vi "FunctDataMgr.Send Local SW Info.vi"(8 "error in (no error)":errorcluster, 11 "FunctDataMgr in":refnum<class "FunctDataMgr.lvclass">) -> (0 "error out":errorcluster, 3 "FunctDataMgr out":refnum<class "FunctDataMgr.lvclass">)   [LabVIEW 2018, in "FunctDataMgr.lvclass"]
uses:
  FunctDataMgr.lvclass
  FunctDataMgr.lvclass/FunctDataMgr.ctl
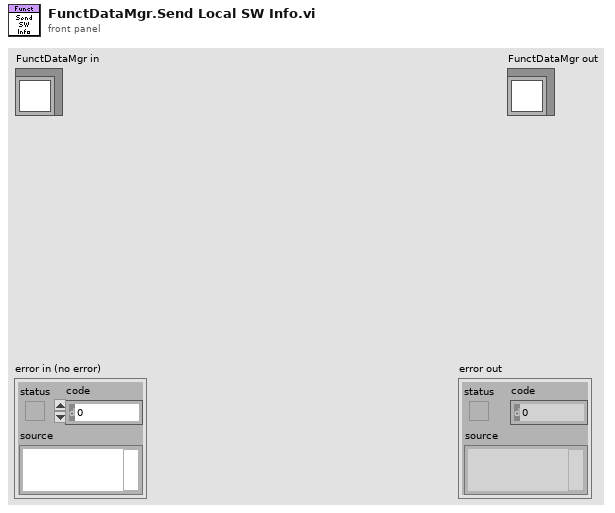
[diagram p1: front panel]
types:
  T1 = typedef "TestResult.SW Item.ctl" = cluster{"Name":string, "PN":string, "Version":string, "Note":string}
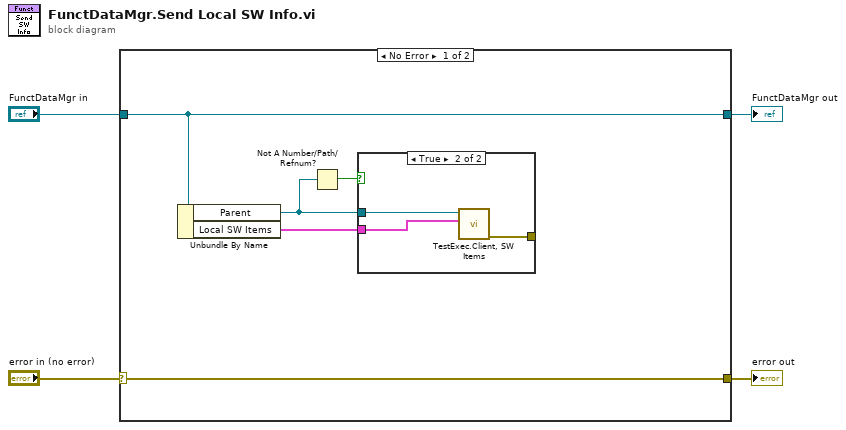
[diagram p0: block diagram]
diagram:
  n1 = case shown="No Error" "error in (no error)" {
    selector: "error in (no error)" -> [w9 w14]
    tunnel: [w9 w14] -> w3
    tunnel: [w8 w13] -> w1
    tunnel: "FunctDataMgr in" -> [w8 w13]
    frame No Error {
      n2 = Unbundle By Name(w8) -> ("Parent"=w6:refnum<queue>, "Local SW Items"=w5:T1[])
      n3 = Not A Number/Path/Refnum?(number/path/refnum=w6) -> (NaN/Path/Refnum?=w7:bool)
      n4 = case shown="True" w7 {
        tunnel: w6 -> [_ w12]
        tunnel: w5 -> [_ w11]
        tunnel: [_ w10] -> _
        frame False {
        }
        frame True {
          n5 = call "TestExec.Client, SW Items.vi"("SW Items"=w11, "Q In"=w12) -> ("error out"=w10:errorcluster)  [unwired: 8 in, 1 out]
        }
      }
    }
    frame Error {
    }
  }
  "error out" <- w3
  "FunctDataMgr out" <- w1
